vi "thcd_set_samp.vi"(4 "thcd_com":T1(ring), 5 "thcd_delay":u32=500, 6 "err_in":errorcluster, 7 "thcd_val":dbl min=0.0 max=99999.0 format="%#.6g", 8 "thcd_ch":T2, 9 "thcd_visa":refnum<visa-resource-name>) -> (0 "err_out":errorcluster, 1 "thcd_st":bool, 2 "thcd_res_msg":string, 3 "thcd_visa":refnum<visa-resource-name>)   [LabVIEW 2018, in "1039_mod.lvlib"]
uses:
  thcd_controls/ctrl_chn_thcd.ctl
  1039_mod/1039_mod.lvlib
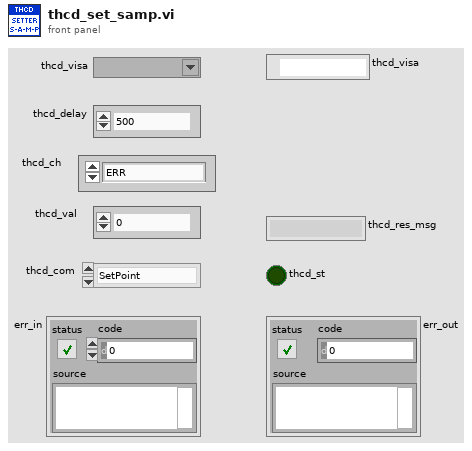
[diagram p1: front panel]
types:
  T1 = enum16{"SetPoint", "AlarmH", "AlarmL", "Multiplier", "CalibValue"}
  T2 = typedef "ctrl_chn_thcd.ctl" = enum8{"ERR", "1", "2", "3", "4"}
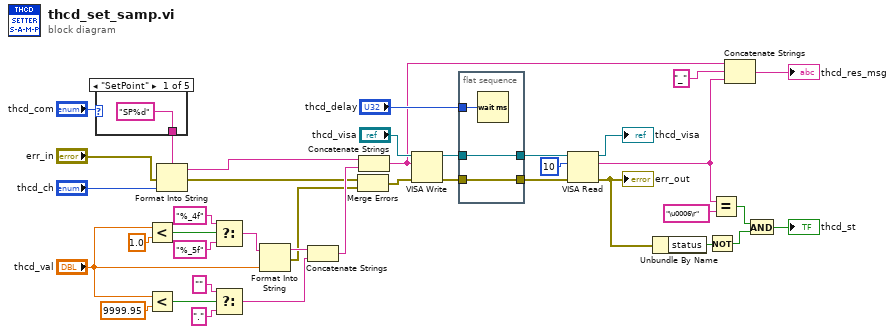
[diagram p0: block diagram]
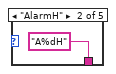
[diagram p2: hidden frame]
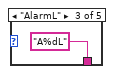
[diagram p3: hidden frame]
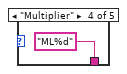
[diagram p4: hidden frame]
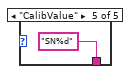
[diagram p5: hidden frame]
diagram:
  n1 = case shown="\"SetPoint\"" "thcd_com" {
    tunnel: ["SP%d" ("format string") "A%dH" ("format string") "A%dL" ("format string") "ML%d" ("format string") "SN%d" ("format string")] -> w33
    frame "SetPoint" {
    }
    frame "AlarmH" {
    }
    frame "AlarmL" {
    }
    frame "Multiplier" {
    }
    frame "CalibValue" {
    }
  }
  n2 = Less?(x="thcd_val", y=1.0) -> (x < y?=w29:bool)
  n3 = Less?(x="thcd_val", y=9999.95) -> (x < y?=w22:bool)
  n4 = Format Into String(format string=w33, error in="err_in", "thcd_ch") -> (resulting string=w19:string, error out=w17:errorcluster)  [unwired: 1 in]
  n5 = Select(t="%_4f" ("format string"), s=w29, f="%_5f" ("format string")) -> (s? t:f=w28:string)
  n6 = Select(t="" ("format string"), s=w22, f="." ("format string")) -> (s? t:f=w21:string)
  n7 = Format Into String(format string=w28, "thcd_val") -> (resulting string=w27:string, error out=w15:errorcluster)  [unwired: 2 in]
  n8 = Concatenate Strings(w27, w21) -> (w18:string)
  n9 = Merge Errors(w17, w15) -> (w16:errorcluster)
  n10 = Concatenate Strings(w19, w18) -> (w3:string)
  n11 = VISA Write(VISA resource name="thcd_visa", write buffer=w3, error in (no error)=w16) -> (VISA resource name out=w38:refnum<visa-resource-name>, error out=w39:errorcluster)  [unwired: 1 out]
  n12 = flat-sequence {
    tunnel: w39 -> [w46]
    tunnel: [w46] -> w6
    tunnel: w38 -> [w45]
    tunnel: [w45] -> w7
    tunnel: "thcd_delay" -> [w47]
    frame #0 {
      n13 = Wait (ms)(milliseconds to wait=w47) -> ()  [unwired: 1 out]
    }
  }
  n14 = VISA Read(VISA resource name=w7, byte count=u32 10, error in (no error)=w6) -> (VISA resource name out=→"thcd_visa":refnum<visa-resource-name>, read buffer=w8:string, error out=w5:errorcluster)  [unwired: 1 out]
  "err_out" <- w5
  n15 = Unbundle By Name(w5) -> ("status"=w14:bool)
  n16 = Not(x=w14) -> (.not. x?=w11:bool)
  n17 = Equal?(x=w8, y="\u0006\r") -> (x = y?=w12:bool)
  n18 = Concatenate Strings(w3, "_", w8) -> (→"thcd_res_msg":string)
  n19 = And(x=w12, y=w11) -> (x .and. y?=→"thcd_st":bool)
